vi "TCP Read com tamanho.vi"(0 "connection ID":refnum<k5>, 5 "error in (no error)":errorcluster) -> (14 "connection out":refnum<k5>, 16 "data out":string, 19 "error out":errorcluster)   [LabVIEW 2012]
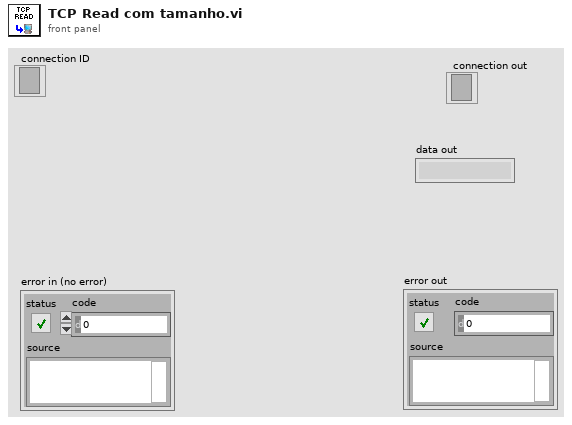
[diagram p1: front panel]
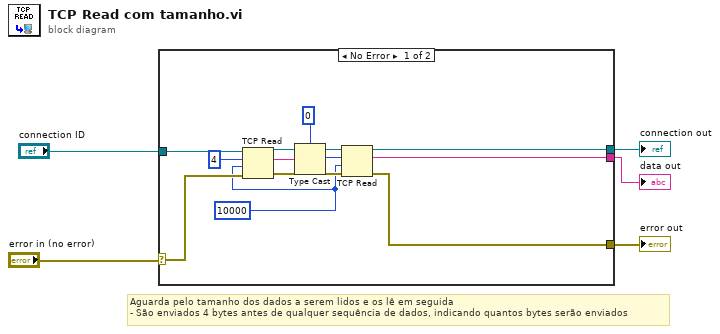
[diagram p0: block diagram]
diagram:
  # "Aguarda pelo tamanho dos dados a serem lidos e os lê em seguida\n- São enviados 4 bytes antes de qualquer sequência de dados, indicando quantos bytes serão enviados"
  n1 = case shown="No Error" "error in (no error)" {
    selector: "error in (no error)" -> [w16 w18]
    tunnel: "connection ID" -> [w17 w19]
    tunnel: [w9 _] -> w2
    tunnel: [w8 w18] -> w3
    tunnel: [w7 w19] -> w1
    frame No Error {
      w6 = 10000 ("timeout ms (25000)")
      n2 = TCP Read(connection ID=w17, bytes to read=4, error in (no error)=w16, 9:w6) -> (connection ID out=w12:refnum<k5>, data out=w14:string, error out=w11:errorcluster)  [unwired: 1 in]
      n3 = Type Cast(type=0, x=w14) -> (*(type *) &x=w10:i32)
      n4 = TCP Read(connection ID=w12, bytes to read=w10, error in (no error)=w11, 9:w6) -> (connection ID out=w7:refnum<k5>, data out=w9:string, error out=w8:errorcluster)  [unwired: 1 in]
    }
    frame Error {
    }
  }
  "error out" <- w3
  "data out" <- w2
  "connection out" <- w1
